vi "Client.vi"(6 "timeout (ms) [500]":i32=500, 8 "error in (no error)":errorcluster, 9 "Data in":variant, 10 "Command in":variant, 11 "Instrument.Aerotech in":refnum<class "Instrument.Aerotech.lvclass">) -> (0 "error out":errorcluster, 1 "Data out":variant, 2 "Command out":string, 3 "Instrument.Aerotech out":refnum<class "Instrument.Aerotech.lvclass">)   [LabVIEW 2019, in "Instrument.Aerotech.lvclass"]
doc: "Remote API call via LocalClient.vi or RemoteClient.vi"
uses:
  Instrument.Aerotech.lvclass
  <userlib>/LevyLab/Instrument Framework/Instrument Types/Delay Line/Typedefs/DelayLine.Commands--Enum.ctl
  <userlib>/LevyLab/Instrument Framework/Instrument Types/Delay Line/Typedefs/DelayLine.setDelay--cluster.ctl
  Instrument.Aerotech.lvclass/Instrument.Aerotech.ctl
  <userlib>/LevyLab/Instrument Framework/Instrument Types/Delay Line/Typedefs/DelayLine.getDelay--cluster.ctl
  Aerotech-Ensemble-LabVIEW/2010-5.6/Motion/MoveAbsSingle.vi
  <userlib>/LevyLab/Instrument Framework/Instrument Types/Delay Line/Instrument.DelayLine.lvclass
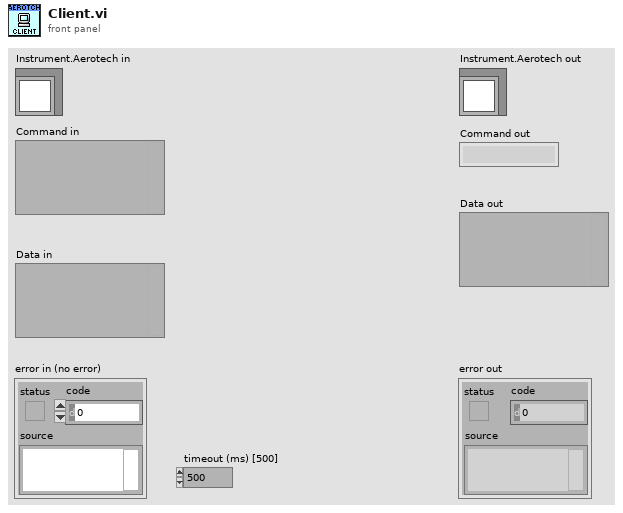
[diagram p1: front panel]
types:
  T1 = typedef "Instrument.DelayLine.lvclass/DelayLine.Commands--Enum.ctl" = enum16{"getDelay", "setDelay"}
  T2 = typedef "Instrument.DelayLine.lvclass/DelayLine.setDelay--cluster.ctl" = cluster{"delay":dbl, "rate":dbl}
  T3 = typedef "Instrument.DelayLine.lvclass/DelayLine.getDelay--cluster.ctl" = cluster{"delay":dbl, "Finished?":bool}
  T4 = typedef "ControllerDiagPacket.ctl" = cluster{"Count":i32, "Packet Time":i64, "Axes":T5[], "error":errorcluster}
  T5 = typedef "AxisDiagPacket.ctl" = cluster{"Axis Name":string, "Acceleration Command":dbl, "Amplifier Temperature":sgl, "Analog Input 0":dbl, "Analog Input 1":dbl, "Analog Output 0":dbl, "Analog Output 1":dbl, "Axis Fault (num)":i32, "Axis Fault (str)":string, "Axis Fault (bits)":cluster{"AmplifierFault":bool, "AmplifierTemperatureFault":bool, "CcwEndOfTravelLimitFault":bool, "CcwSoftwareLimitFault":bool, "CommunicationLostFault":bool, "CwEndOfTravelLimitFault":bool, "CwSoftwareLimitFault":bool, "EmergencyStopFault":bool, "EncoderFault":bool, "ExternalFault":bool, "FeedbackScalingFault":bool, "HallSensorFault":bool, "MarkerSearchFault":bool, "MaxVelocityCommandFault":bool, "MotorTemperatureFault":bool, "None":bool, "OverCurrentFault":bool, "PositionErrorFault":bool, "PositionFeedbackFault":bool, "PowerSupplyFault":bool, "VelocityErrorFault":bool, "VelocityFeedbackFault":bool, "VoltageClampFault":bool}, "Axis Status (num)":i32, "Axis Status (str)":string, "Axis Status (bits)":cluster{"AccelerationPhase":bool, "AutofocusActive":bool, "BrakeOutput":bool, "CalibrationActive":bool, "CalibrationEnabled":bool, "CcwEndOfTravelLimitInput":bool, "CommandShapingFilterDone":bool, "CosineEncoderError":bool, "CurrentClamp":bool, "CwEndOfTravelLimitInput":bool, "DecelerationPhase":bool, "EmergencyStopInput":bool, "Enabled":bool, "GantryMasterActive":bool, "GantryModeActive":bool, "HallAInput":bool, "HallBInput":bool, "HallCInput":bool, "Homed":bool, "HomeLimitInput":bool, "Homing":bool, "InPosition":bool, "InPosition2":bool, "JoystickControl":bool, "MarkerInput":bool, "MasterMotionSuppressed":bool, "MasterSlaveControl":bool, "MotionIsCw":bool, "MoveActive":bool, "None":bool, "PositionCaptureActive":bool, "ServoControl":bool, "SineEncoderError":bool}, "Current Command":sgl, "Current Error":sgl, "Current Feedback":sgl, "Digital Input 0":i32, "Digital Input 1":i32, "Digital Input 2":i32, "Digital Output 0":i32, "Digital Output 1":i32, "Digital Output 2":i32, "Position Feedback Auxiliary":dbl, "Position Command":dbl, "Position Error":dbl, "Position Feedback":dbl, "Program Position Command":dbl, "Program Position Error":dbl, "Program Position Feedback":dbl, "Velocity Command":dbl, "Velocity Error":dbl, "Velocity Feedback":dbl}
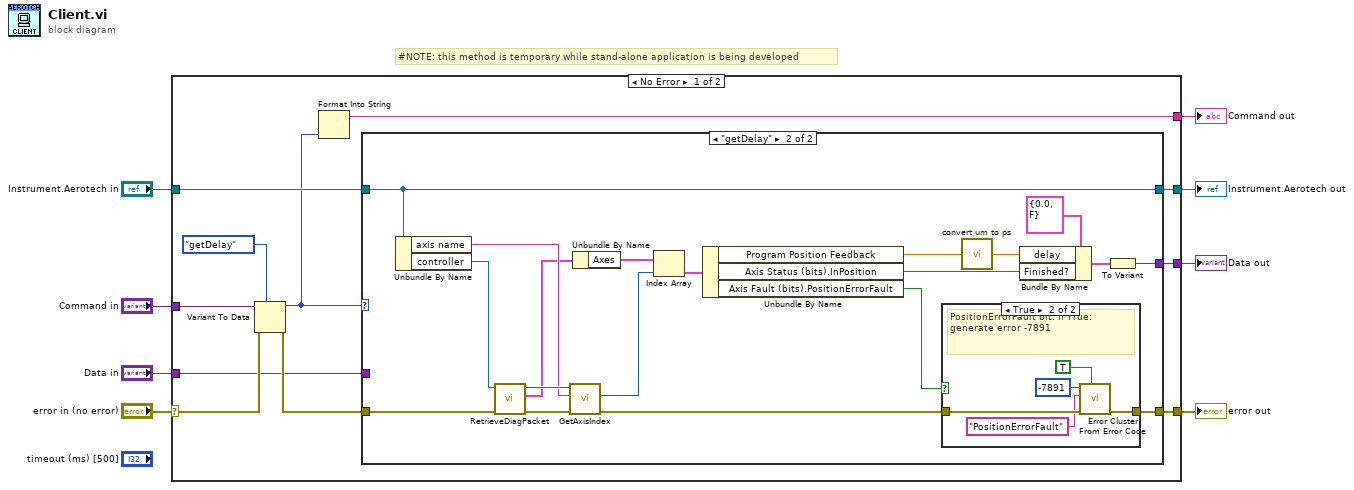
[diagram p0: block diagram]
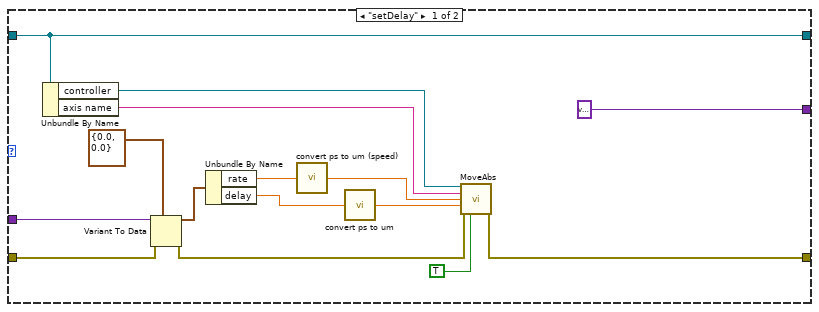
[diagram p2: hidden frame]
diagram:
  # "#NOTE: this method is temporary while stand-alone application is being developed"
  n1 = case shown="No Error" "error in (no error)" {
    selector: "error in (no error)" -> [w11 w61]
    tunnel: "Instrument.Aerotech in" -> [w19 w60]
    tunnel: [w18 w60] -> w7
    tunnel: [w17 w61] -> w6
    tunnel: "Command in" -> [w16 _]
    tunnel: "Data in" -> [w9 _]
    tunnel: [w15 _] -> w3
    tunnel: [w13 _] -> w2
    frame No Error {
      n2 = Variant To Data(error in=w11, type=DelayLine.Commands--Enum."getDelay" ("command"), Variant=w16) -> (data=w14:T1, error out=w10:errorcluster)
      n3 = Format Into String(w14) -> (resulting string=w13:string)  [unwired: 3 in, 1 out]
      n4 = case shown="\"getDelay\"" w14 {
        tunnel: w10 -> [w24 w46]
        tunnel: w19 -> [w29 w45]
        tunnel: [w29 w45] -> w18
        tunnel: [w28 w44] -> w17
        tunnel: w9 -> [w26 _]
        tunnel: [variant ("Variant") w39] -> w15
        frame "setDelay" {
          n5 = Unbundle By Name(w29) -> ("controller"=w33:refnum<k24>, "axis name"=w32:string)
          n6 = Variant To Data(error in=w24, type=T2 {"delay"=0.0, "rate"=0.0} ("setDelay"), Variant=w26) -> (data=w21:T2, error out=w25:errorcluster)
          n7 = Unbundle By Name(w21) -> ("rate"=w22:dbl, "delay"=w20:dbl)
          n8 = call "convert ps to um (speed).vi"("Delay speed (ps/s)"=w22) -> ("Position speed (um/s)"=w31:dbl)
          n9 = call "convert ps to um.vi"("Delay (ps)"=w20) -> ("Position (um)"=w30:dbl)
          n10 = call-poly "MoveAbs.vi"("controller in"=w33, "axis name"=w32, "speed"=w31, "distance"=w30, "error in (no error)"=w25, "return immediately"=TRUE) -> ("error out"=w28:errorcluster)  [unwired: 8 in, 1 out]
        }
        frame "getDelay" {
          n11 = Unbundle By Name(w45) -> ("axis name"=w38:string, "controller"=w49:refnum<k24>)
          n12 = call "RetrieveDiagPacket.vi"("error in (no error)"=w46, "Controller In"=w49) -> ("error out"=w52:errorcluster, "ControllerDiagPacket"=w36:T4, "Controller Out"=w53:refnum<k24>)  [unwired: 7 in]
          n13 = call "GetAxisIndex.vi"("error in (no error)"=w52, "axis name"=w38, "controller in"=w53) -> ("error out"=w47:errorcluster, "axis index"=w35:i32)  [unwired: 6 in, 1 out]
          n14 = Unbundle By Name(w36) -> ("Axes"=w51:T5[])
          n15 = Index Array(array=w51, index=w35) -> (element=w50:T5)
          n16 = Unbundle By Name(w50) -> ("Program Position Feedback"=w48:dbl, "Axis Status (bits).InPosition"=w41:bool, "Axis Fault (bits).PositionErrorFault"=w37:bool)
          n17 = case shown="True" w37 {
            tunnel: w47 -> [w54 w59]
            tunnel: [w54 w58] -> w44
            frame False {
            }
            frame True {
              # "PositionErrorFault bit. If True: generate error -7891"
              n18 = call <vilib>:"Error Cluster From Error Code.vi"("show call chain? (False)"=TRUE, "error in (no error)"=w59, "error message (\"\")"="PositionErrorFault" ("error message (\"\")"), "error code (0)"=-7891) -> ("error out"=w58:errorcluster)  [unwired: 5 in]
            }
          }
          n19 = call "convert um to ps.vi"("Position (um)"=w48) -> ("Delay (ps)"=w42:dbl)
          n20 = Bundle By Name(cluster=T3 {"delay"=0.0, "Finished?"=FALSE} ("getDelay"), "delay"=w42, "Finished?"=w41) -> (w40:T3)
          n21 = To Variant(anything=w40) -> (Variant=w39:variant)
        }
      }
    }
    frame Error {
    }
  }
  "error out" <- w6
  "Instrument.Aerotech out" <- w7
  "Data out" <- w3
  "Command out" <- w2
